vi "Remove leading and trailing slashes.vi"(1 "string in":string) -> (0 "string out":string)   [LabVIEW 2019, in "LV-Data.AWS CLI.lvclass"]
uses:
  LV-Data.AWS CLI.lvclass
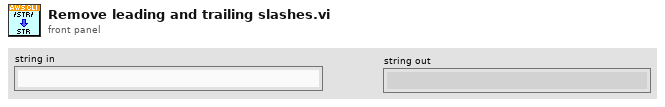
[diagram p1: front panel]
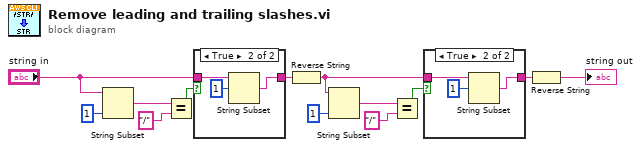
[diagram p0: block diagram]
diagram:
  n1 = String Subset(string="string in", length (rest)=1 ("length (rest)")) -> (substring=w2:string)  [unwired: 1 in]
  n2 = Equal?(x=w2, y="/") -> (x = y?=w4:bool)
  n3 = case shown="True" w4 {
    tunnel: "string in" -> [w14 w17]
    tunnel: [w14 w16] -> w5
    frame False {
    }
    frame True {
      n4 = String Subset(string=w17, offset (0)=1) -> (substring=w16:string)  [unwired: 1 in]
    }
  }
  n5 = Reverse String(1:w5) -> (0:w13:string)
  n6 = String Subset(string=w13, length (rest)=1 ("length (rest)")) -> (substring=w9:string)  [unwired: 1 in]
  n7 = Equal?(x=w9, y="/") -> (x = y?=w7:bool)
  n8 = case shown="True" w7 {
    tunnel: w13 -> [w18 w21]
    tunnel: [w18 w20] -> w6
    frame False {
    }
    frame True {
      n9 = String Subset(string=w21, offset (0)=1) -> (substring=w20:string)  [unwired: 1 in]
    }
  }
  n10 = Reverse String(1:w6) -> (0:→"string out":string)
